vi "TDMs Group&Channel Name.vi"(7 "Ini?":bool, 8 "error in (no error)":errorcluster caption="错误输入（无错误）", 9 "Channel":string[](array[string]), 10 "Group":string[](array[string])) -> (0 "error out":errorcluster caption="错误输出", 1 "Channel":string[](array[string]), 2 "Group":string[](array[string]))   [LabVIEW 2012]
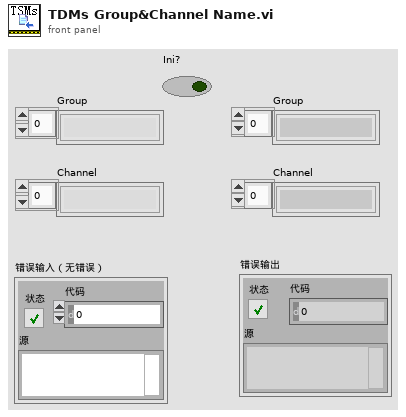
[diagram p1: front panel]
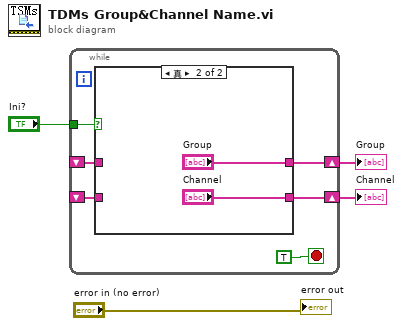
[diagram p0: block diagram]
diagram:
  n1 = while {
    tunnel: "Ini?" -> [w9]
    shift-right: [w8] -> w2
    shift-left: _ -> [w6]
    shift-right: [w7] -> w1
    shift-left: _ -> [w5]
    stop <- TRUE stop-if-true
    n2 = case shown="真" w9 {
      tunnel: [w12 "Group"] -> w8
      tunnel: [w11 "Channel"] -> w7
      tunnel: w6 -> [w12 _]
      tunnel: w5 -> [w11 _]
      frame False {
      }
      frame True {
      }
    }
  }
  "Group" <- w2
  "Channel" <- w1
  "error out" <- "error in (no error)"
